vi "niScope test.vi"() -> ()   [LabVIEW 2013]
uses:
  <instrlib>/niScope/Controls/niScope export destinations.ctl
  <instrlib>/niScope/Controls/niScope exportable signals.ctl
  drivers/niScope/niScope Reference Clock.ctl
  drivers/niScope/niScope Virtual Digitizer.lvlib
panel:
  out "error out":errorcluster
  in  "resource name":refnum<k15>="DAQ::1"
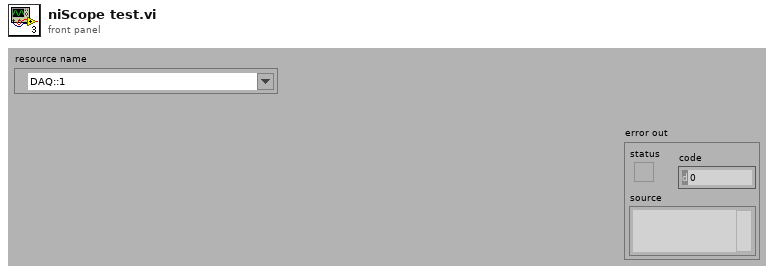
[diagram p1: front panel]
types:
  T1 = typedef "niScope Virtual Digitizer.lvlib/niScope Reference Clock.ctl" = enum16{"VAL_NO_SOURCE", "VAL_CLK_IN", "VAL_PXI_CLOCK", "VAL_EXTERNAL"}
  T2 = typedef "niScope exportable signals.ctl" = u16
  T3 = typedef "niScope export destinations.ctl" = string
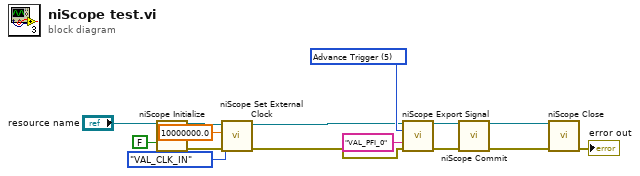
[diagram p0: block diagram]
diagram:
  w11 = T2 5 items=["None"=0, "Start Trigger"=2, "Advance Trigger"=5, "Reference Trigger"=1, "End of Record Event"=4, "End of Acquisition Event"=3, "Ready for Start Event"=7, "Ready for Advance Event"=6, "Ready for Reference Event"=10, "Reference Clock"=100, "Sample Clock"=101, "5 Volt Power"=13] ("signal")
  n1 = call <instrlib>:"niScope Initialize.vi"("resource name"="resource name", "reset device"=FALSE) -> ("instrument handle"=w5:refnum<k15>, "error out"=w6:errorcluster)  [unwired: 12 in]
  n2 = call "niScope Set External Clock.vi"("error in"=w6, "clock source"=niScope_Reference_Clock."VAL_CLK_IN", "ref. clock rate [Hz] (0: use internal clock)"=10000000.0, "niScope reference in"=w5) -> ("error out"=w3:errorcluster, "reference out"=w4:refnum<k15>)  [unwired: 3 in, 3 out]
  n3 = call <instrlib>:"niScope Export Signal.vi"("instrument handle"=w4, "signal"=w11, "output terminal"=T3 "VAL_PFI_0", "error in"=w3) -> ("instrument handle out"=w8:refnum<k15>, "error out"=w10:errorcluster)  [unwired: 10 in]
  n4 = call <instrlib>:"niScope Commit.vi"("instrument handle"=w8, "error in"=w10) -> ("instrument handle out"=w7:refnum<k15>, "error out"=w9:errorcluster)  [unwired: 12 in]
  n5 = call <instrlib>:"niScope Close.vi"("instrument handle"=w7, "error in"=w9) -> ("error out"=→"error out":errorcluster)  [unwired: 13 in]
